vi "Prune.vi"(4 "Delete All Excessive":bool, 6 "File Extension":string="csv", 8 "Error In":errorcluster, 10 "Maximum File Count":i32, 11 "File In":refnum<file>) -> (0 "Error Out":errorcluster, 3 "File Out":refnum<file>)   [LabVIEW 2025, in "LOGlib_LV2025.lvlib" / "File.lvlib"]
uses:
  File.lvlib
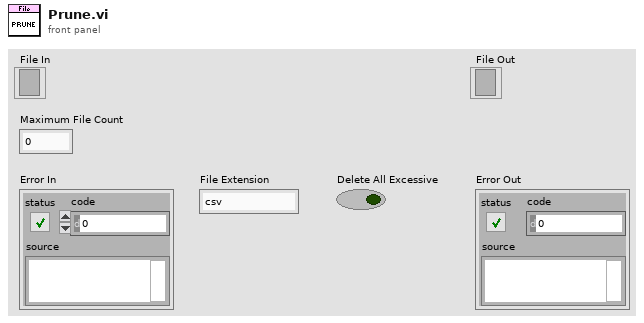
[diagram p1: front panel]
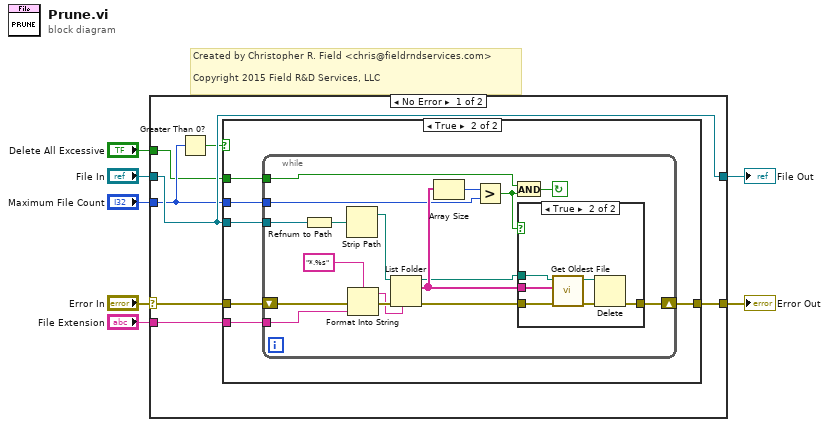
[diagram p0: block diagram]
diagram:
  # "Created by Christopher R. Field <chris@fieldrndservices.com>\n\nCopyright 2015 Field R&D Services, LLC"
  n1 = case shown="No Error" "Error In" {
    selector: "Error In" -> [w14 w47]
    tunnel: "File In" -> [w12 w46]
    tunnel: "Maximum File Count" -> [w11 _]
    tunnel: [w13 w47] -> w4
    tunnel: [w12 w46] -> w3
    tunnel: "File Extension" -> [w9 _]
    tunnel: "Delete All Excessive" -> [w8 _]
    frame No Error {
      n2 = Greater Than 0?(x=w11) -> (x > 0?=w10:bool)
      n3 = case shown="True" w10 {
        tunnel: w14 -> [w15 w21]
        tunnel: w11 -> [_ w17]
        tunnel: [w15 w20] -> w13
        tunnel: w12 -> [_ w19]
        tunnel: w9 -> [_ w18]
        tunnel: w8 -> [_ w16]
        frame False {
        }
        frame True {
          n4 = while {
            tunnel: w19 -> [w31]
            tunnel: w18 -> [w27]
            tunnel: w17 -> [w25]
            shift-right: [w32] -> w20
            shift-left: w21 -> [w36]
            tunnel: w16 -> [w22]
            stop <- w23 continue-if-true
            n5 = Refnum to Path(1:w31) -> (0:w38:path)
            n6 = Strip Path(path=w38) -> (stripped path=w37:path)  [unwired: 1 out]
            n7 = Format Into String(format string="*.%s", error in=w36, w27) -> (resulting string=w28:string, error out=w30:errorcluster)  [unwired: 1 in]
            n8 = List Folder(path=w37, pattern=w28, error in=w30) -> (path out=w33:path, filenames=w34:string[], error out=w35:errorcluster)  [unwired: 1 in, 1 out]
            n9 = Array Size(array=w34) -> (size(s)=w26:i32)
            n10 = Greater?(x=w26, y=w25) -> (0:w24:bool)
            n11 = And(x=w22, y=w24) -> (x .and. y?=w23:bool)
            n12 = case shown="True" w24 {
              tunnel: w35 -> [w39 w45]
              tunnel: w34 -> [_ w43]
              tunnel: w33 -> [_ w44]
              tunnel: [w39 w42] -> w32
              frame False {
              }
              frame True {
                n13 = call "Get Oldest File.vi"("Error In"=w45, "File Names"=w43, "Folder"=w44) -> ("Error Out"=w40:errorcluster, "Oldest File"=w41:path)  [unwired: 7 in]
                n14 = Delete(path (use dialog)=w41, error in=w40) -> (error out=w42:errorcluster)  [unwired: 3 in, 2 out]
              }
            }
          }
        }
      }
    }
    frame Error {
    }
  }
  "Error Out" <- w4
  "File Out" <- w3
